vi "find_sub_contour.vi"(10 "Segment Information":T1(array[cluster]), 11 "Y Resolution":i32) -> (2 "Y":dbl[](array[numeric]), 3 "X":dbl[](array[numeric]))   [LabVIEW 2017]
panel:
  out "max corner":dbl[][](array[numeric])
  in  "max index":dbl
  in  "max area":dbl
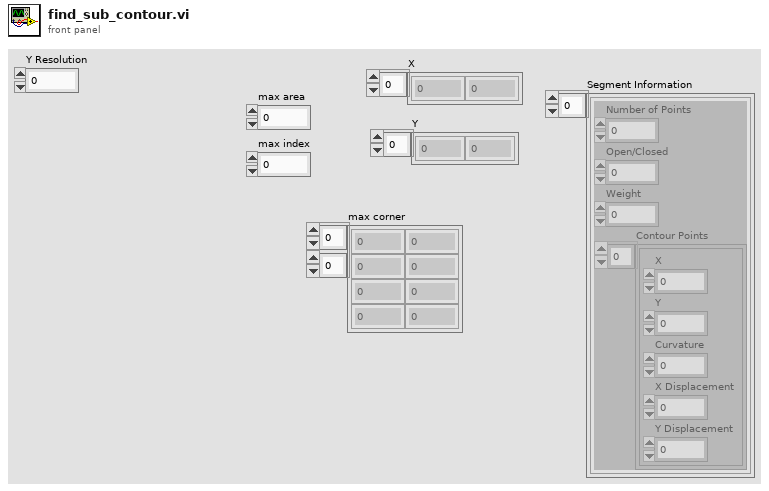
[diagram p1: front panel]
types:
  T1 = cluster{"Number of Points":i32, "Open/Closed":i32, "Weight":dbl, "Contour Points":cluster{"X":dbl, "Y":dbl, "Curvature":dbl, "X Displacement":dbl, "Y Displacement":dbl}[]}[]
  T2 = cluster{"X":dbl, "Y":dbl, "Curvature":dbl, "X Displacement":dbl, "Y Displacement":dbl}[]
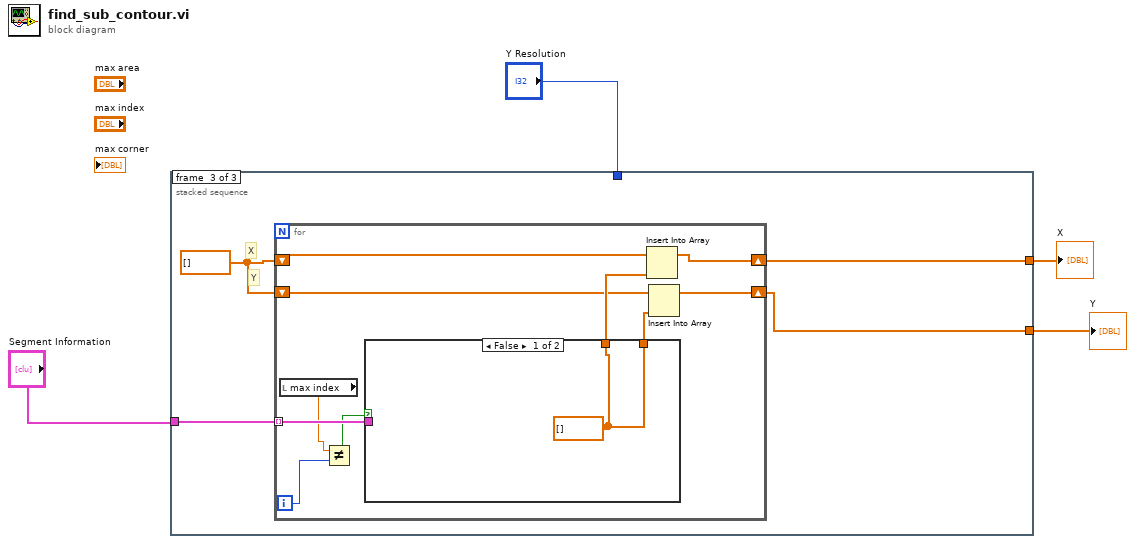
[diagram p0: block diagram]
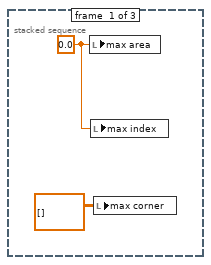
[diagram p2: hidden frame]
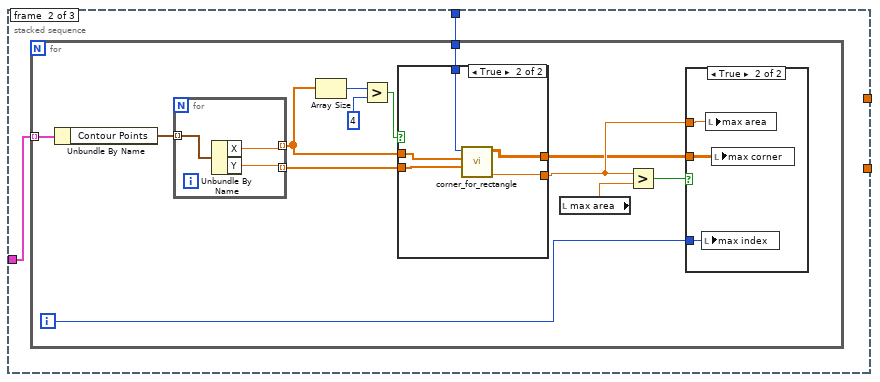
[diagram p3: hidden frame]
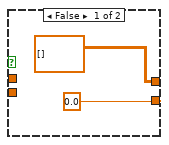
[diagram p5: hidden frame]
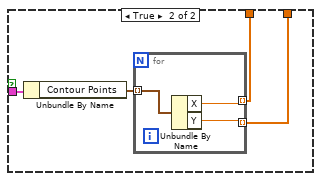
[diagram p6: hidden frame]
diagram:
  n1 = stacked-sequence {
    tunnel: "Y Resolution" -> [_ w8 _]
    tunnel: "Segment Information" -> [_ w7 w38]
    tunnel: [_ _ w36] -> w2
    tunnel: [_ _ w35] -> w1
    frame #0 {
      w6 = 0.0
      n2 = local write "max area"(w6) -> ()
      n3 = local write "max index"(w6) -> ()
      n4 = local write "max corner"(dbl[][] [] ("max corner")) -> ()
    }
    frame #1 {
      n5 = for {
        tunnel: w7 -> [w21] mode=indexing
        tunnel: w8 -> [w14]
        i -> [w10]
        n6 = Unbundle By Name(w21) -> ("Contour Points"=w20:T2)
        n7 = for {
          tunnel: w20 -> [w34] mode=indexing
          tunnel: [w33] -> w16 mode=indexing
          tunnel: [w32] -> w15 mode=indexing
          n8 = Unbundle By Name(w34) -> ("X"=w33:dbl, "Y"=w32:dbl)
        }
        n9 = Array Size(array=w16) -> (size(s)=w19:i32)
        n10 = Greater?(x=w19, y=4) -> (0:w17:bool)
        n11 = case shown="True" w17 {
          tunnel: w16 -> [_ w31]
          tunnel: w15 -> [_ w30]
          tunnel: w14 -> [_ w29]
          tunnel: [0.0 w28] -> w11
          tunnel: [dbl[][] [] ("max corner") w27] -> w9
          frame False {
          }
          frame True {
            n12 = call "corner_for_rectangle.vi"("Y"=w30, "X"=w31, "Y Resolution"=w29) -> ("area"=w28:dbl, "corner"=w27:dbl[][])  [unwired: 7 in]
          }
        }
        n13 = local read "max area"() -> (w13:dbl)
        n14 = Greater?(x=w11, y=w13) -> (0:w12:bool)
        n15 = case shown="True" w12 {
          tunnel: w11 -> [_ w24]
          tunnel: w10 -> [_ w23]
          tunnel: w9 -> [_ w22]
          frame False {
          }
          frame True {
            n16 = local write "max index"(w23) -> ()
            n17 = local write "max area"(w24) -> ()
            n18 = local write "max corner"(w22) -> ()
          }
        }
      }
    }
    frame #2 {
      w37 = dbl[] []
      # "Y"
      # "X"
      n19 = for {
        tunnel: w38 -> [w48] mode=indexing
        shift-right: [w45] -> w36
        shift-left: w37 -> [w47]
        shift-right: [w42] -> w35
        shift-left: w37 -> [w44]
        i -> [w39]
        n20 = local read "max index"() -> (w40:dbl)
        n21 = Not Equal?(x=w40, y=w39) -> (x != y?=w41:bool)
        n22 = case shown="False" w41 {
          tunnel: w48 -> [_ w52]
          tunnel: [w49 w51] -> w46
          tunnel: [w49 w50] -> w43
          frame False {
            w49 = dbl[] []
          }
          frame True {
            n23 = Unbundle By Name(w52) -> ("Contour Points"=w53:T2)
            n24 = for {
              tunnel: w53 -> [w56] mode=indexing
              tunnel: [w55] -> w51 mode=indexing
              tunnel: [w54] -> w50 mode=indexing
              n25 = Unbundle By Name(w56) -> ("X"=w55:dbl, "Y"=w54:dbl)
            }
          }
        }
        n26 = Insert Into Array(array=w47, new element=w46) -> (w45:dbl[])  [unwired: 1 in]
        n27 = Insert Into Array(array=w44, new element=w43) -> (w42:dbl[])  [unwired: 1 in]
      }
    }
  }
  "X" <- w2
  "Y" <- w1
